vi "Example_Main.vi"() -> ()   [LabVIEW 2018, in "HttpExamples.lvlib"]
doc: "<b> </b> <b> </b>\nHttpClient_NET\nJustin Young - Viviota\nCopyright (c) 2021\nLicense: BSD"
uses:
  HttpExamples.lvlib
  Types/method_enum.ctl
  Types/ContentType.ctl
  <vilib>/Utility/sysdir.llb/System Directory Type.ctl
  HttpDownloadTask/HttpDownloadTask.lvclass/HttpDownloadTask.ctl
  HttpDownloadTask/Accessors/Read HttpResponseMessage.vi
  HttpContent_string/HttpContent_String.lvclass
  C:/Viviota/Projects/R&D/__OpenSource/VIV_HTTP_REST_NET/HttpContent/HttpContent.lvclass
  HttpHeaders_content/HttpHeaders_Content.lvclass
  C:/Viviota/Projects/R&D/__OpenSource/VIV_HTTP_REST_NET/HTTPHeaders_NET/HttpHeaders_NET.lvclass
  HttpHeaders_Request/HttpHeaders_Request.lvclass
  HttpHeaders_response/HttpHeaders_Response.lvclass
  <vilib>/httpClient/Base64Encode.vi
  HttpResponseMessage/HttpResponseMessage.lvclass
  HTTPHeaders_NET/HttpHeaders_NET.lvclass
  LabVIEWHTTPClient_NET/HttpClient_NET.lvclass
  WebProxy_NET/WebProxy_NET.lvclass
  HttpClient_NET.lvlib
  HttpRequestMessage/HttpRequestMessage.lvclass
  HttpContent_ByteArray/HttpContent_ByteArray.lvclass
  HttpContent_Stream/HttpContent_Stream.lvclass
  HttpContent_Multipart/HttpContent_Multipart.lvclass
  HttpContent/HttpContent.lvclass
  HttpDownloadTask/HttpDownloadTask.lvclass
panel:
  out "Error Out":errorcluster
  out "Status":u32
  in  "ExecutionExample":T1(ring)
  out "Header Values":string[](array[string])
  out "Header Names":string[](array[string])
  out "Response":string
  out "StatusCode":i32(ring)=100 items=["Continue"=100, "SwitchingProtocols"=101, "OK"=200, "Created"=201, "Accepted"=202, "NonAuthoritativeInformation"=203, "NoContent"=204, "ResetContent"=205, "PartialContent"=206, "MultipleChoices, Ambiguous"=300, "MovedPermanently, Moved"=301, "Found, Redirect"=302, "SeeOther, RedirectMethod"=303, "NotModified"=304, "UseProxy"=305, "Unused"=306, "TemporaryRedirect, RedirectKeepVerb"=307, "BadRequest"=400, "Unauthorized"=401, "PaymentRequired"=402, "Forbidden"=403, "NotFound"=404, "MethodNotAllowed"=405, "NotAcceptable"=406, "ProxyAuthenticationRequired"=407, "RequestTimeout"=408, "Conflict"=409, "Gone"=410, "LengthRequired"=411, "PreconditionFailed"=412, "RequestEntityTooLarge"=413, "RequestUriTooLong"=414, "UnsupportedMediaType"=415, "RequestedRangeNotSatisfiable"=416, "ExpectationFailed"=417, "UpgradeRequired"=426, "InternalServerError"=500, "NotImplemented"=501, "BadGateway"=502, "ServiceUnavailable"=503, "GatewayTimeout"=504, "HttpVersionNotSupported"=505]
  out "ReasonPhrase":string
  out "Timeout":bool
  in  "URL":string="https://reqres.in/api/users?page=2"
  in  "ProxyPort":i32=443
  in  "ProxyHost":string
  in  "UseProxy":bool
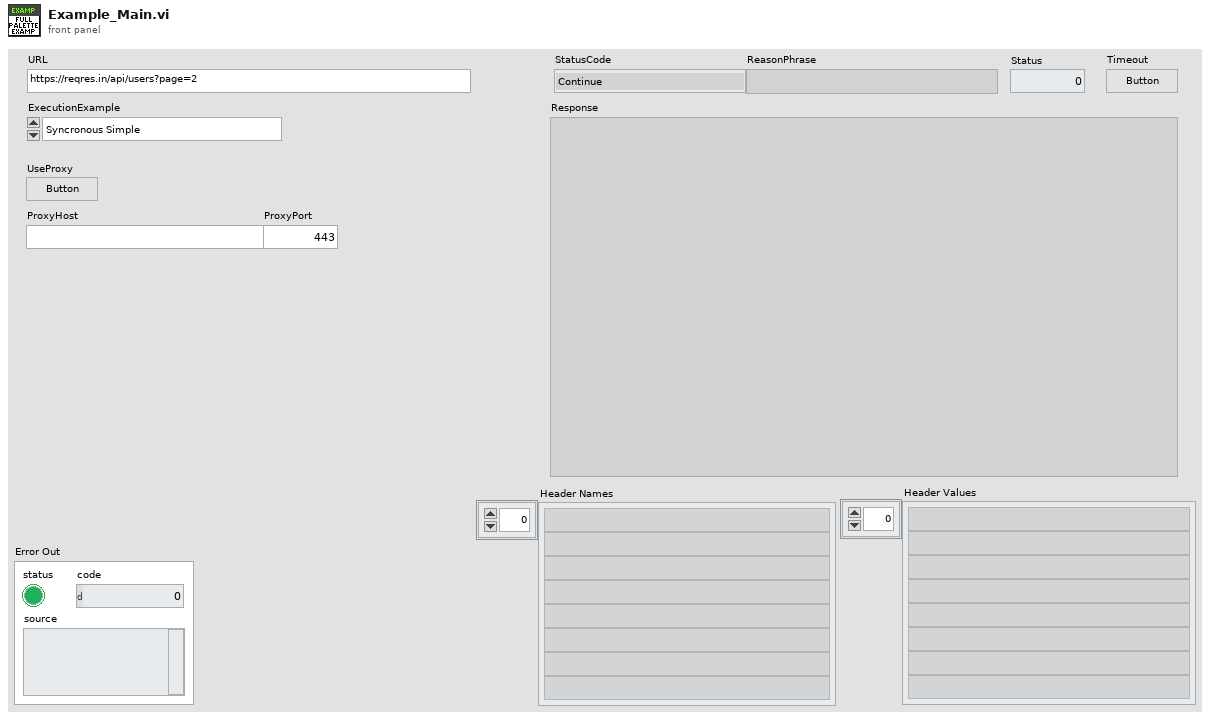
[diagram p1: front panel]
types:
  T1 = enum16{"Syncronous Simple", "Syncronous Advanced", "Asyncronous", "Asyncronous Queue", "Asyncronous File Download"}
  T2 = typedef "HttpClient_NET.lvlib/ContentType.ctl" = string
  T3 = enum16{"String", "ByteArray", "File", "MultiPart"}
  T4 = typedef "HttpClient_NET.lvlib/method_enum.ctl" = enum16{"GET", "PUT", "POST", "DELETE", "HEAD", "TRACE", "SEND"}
  T5 = typedef "HttpClient_NET.lvlib/ResponseHeaders_Cluster.ctl" = cluster{"ResponseHeader":refnum<class "HttpHeaders_Response.lvclass">, "ContentHeaders":refnum<class "HttpHeaders_Content.lvclass">}
  T6 = cluster{"HTTPHeaders_NET out":refnum<class "HttpHeaders_Response.lvclass">, "HTTPHeaders":refnum<class "HttpHeaders_Content.lvclass">}
  T7 = typedef "System Directory Type.ctl" = i32
  T8 = typedef "HttpClient_NET.lvlib/HttpDownloadTask.lvclass/DownloadTask_ref.ctl" = refnum<data-value>
  T9 = typedef "HttpClient_NET.lvlib/DownloadStats_Cluster.ctl" = cluster{"PositionCurrent":dbl, "PositionPrev":dbl, "TimeCurrent":timestamp, "TimePrev":timestamp, "TimeTotal":dbl, "PositionTotal":dbl, "TimeArray":dbl[], "PositionDifArray":dbl[], "CurrentRate":dbl, "RunningRate_10":dbl, "RunningRate":dbl, "Length":dbl}
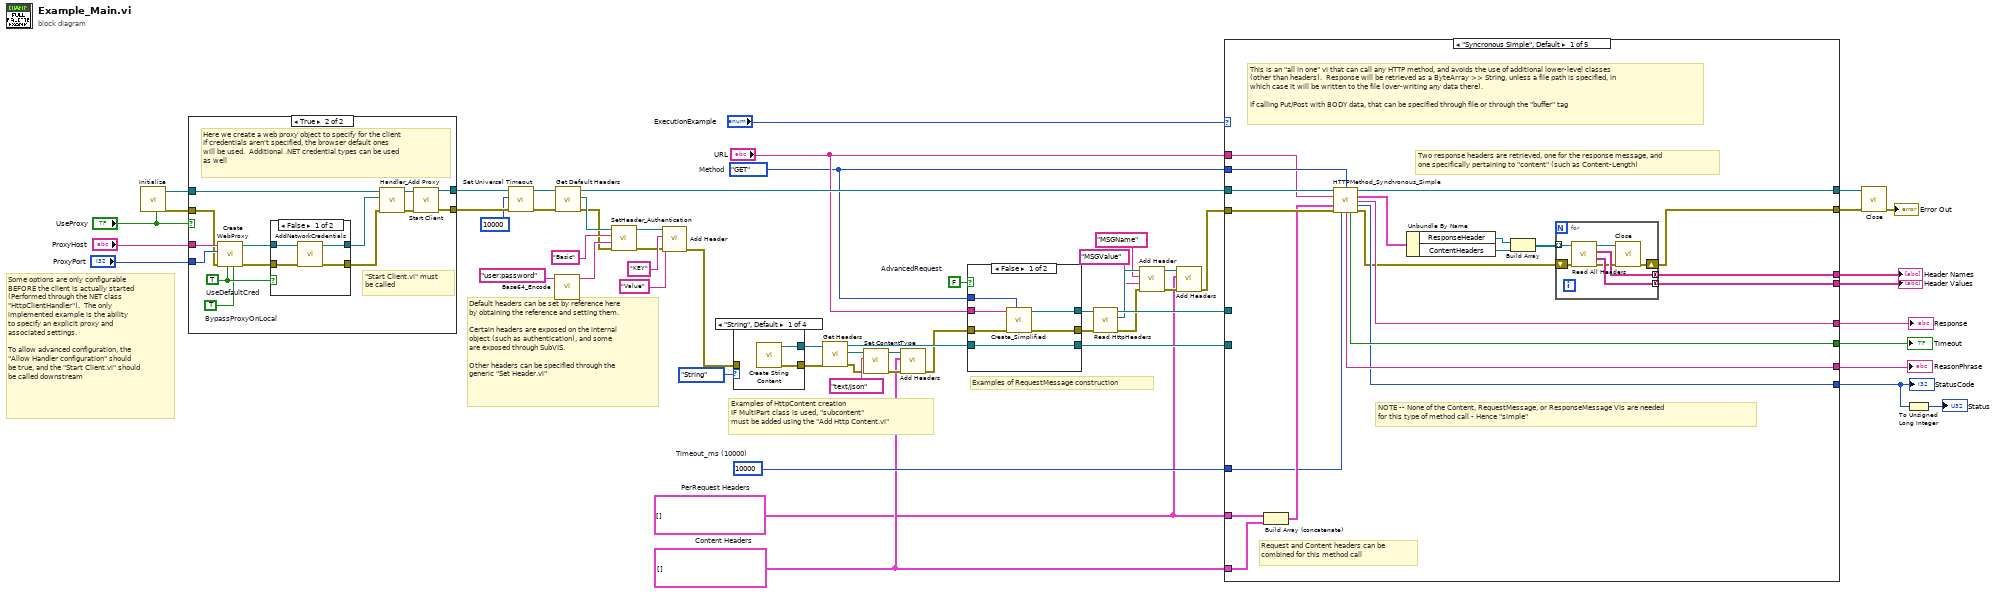
[diagram p0: block diagram]
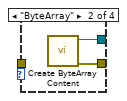
[diagram p4: hidden frame]
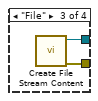
[diagram p5: hidden frame]
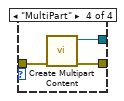
[diagram p6: hidden frame]
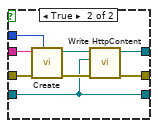
[diagram p7: hidden frame]
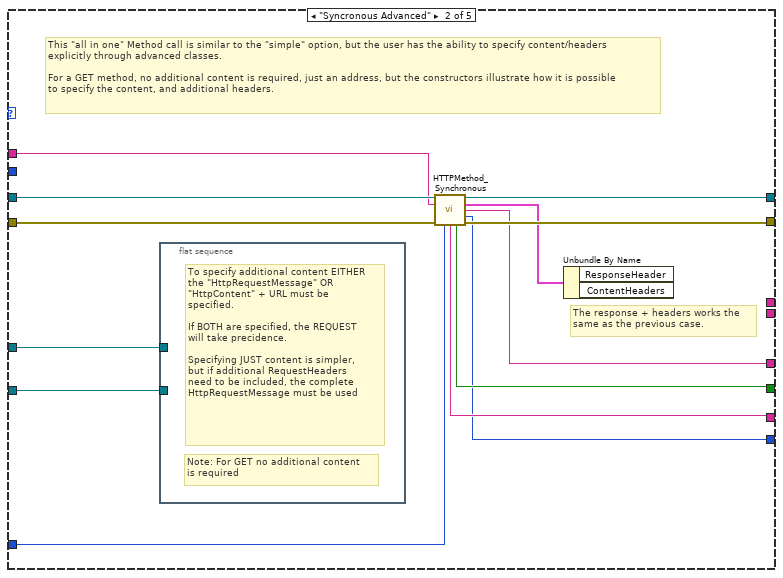
[diagram p8: hidden frame]
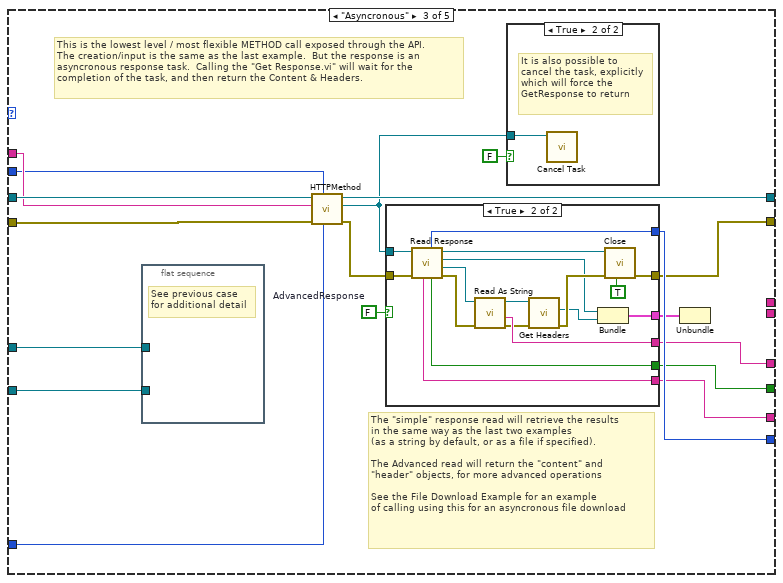
[diagram p9: hidden frame]
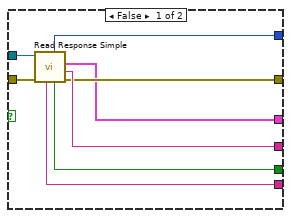
[diagram p11: hidden frame]
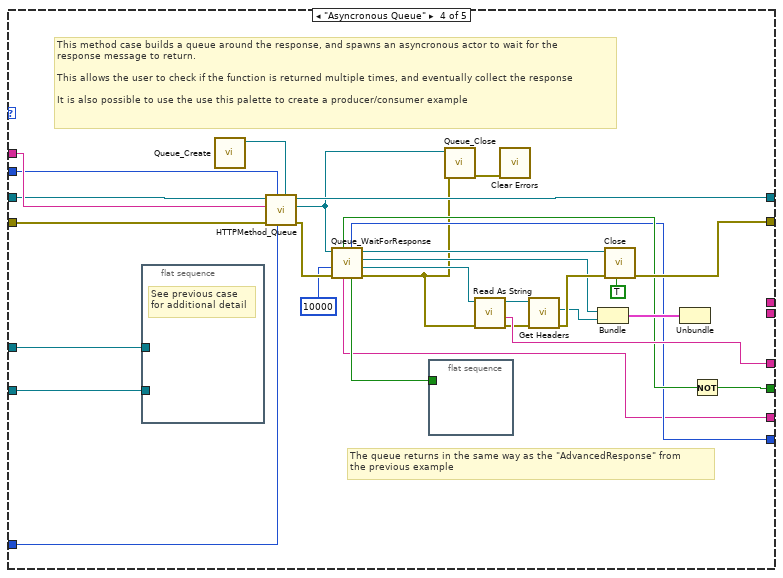
[diagram p12: hidden frame]
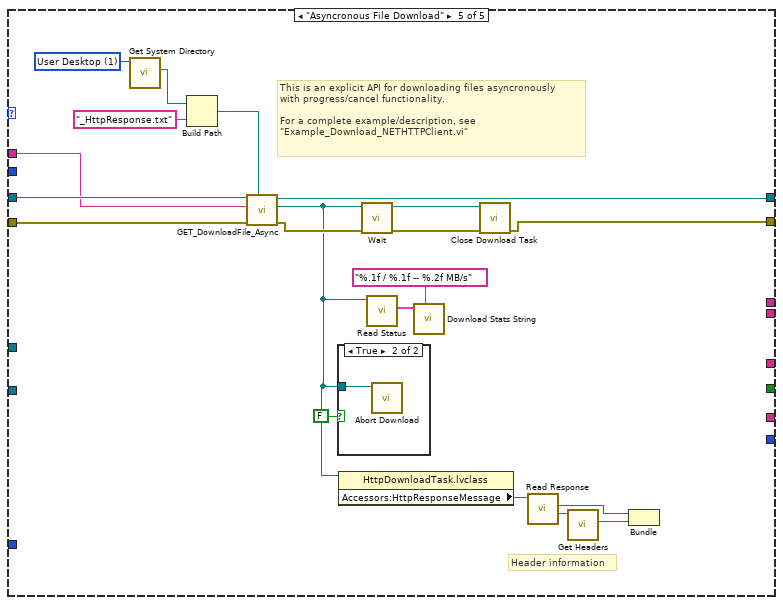
[diagram p13: hidden frame]
diagram:
  w12 = FALSE  # AdvancedRequest
  w38 = 10000  # Timeout_ms (10000)
  w5 = cluster{"header":string, "value":string}[] []  # Content Headers
  w4 = cluster{"header":string, "value":string}[] []  # PerRequest Headers
  w29 = method_enum."GET"  # Method
  # "Examples of HttpContent creation\nIF MultiPart class is used, \"subcontent\"\nmust be added using the \"Add Http Content.vi\""
  # "Examples of RequestMessage construction"
  # "Default headers can be set by reference here\nby obtaining the reference and setting them.\n\nCertain headers are exposed on the internal\nobject (such as authentication), and some\nare exposed through SubVIS.\n\nOther headers can be specified through the \ngeneric \"Set Header.vi\""
  # "Some options are only configurable\nBEFORE the client is actually started\n(Performed through the NET class\n\"HttpClientHandler\").  The only\nimplemented example is the ability\nto specify an explicit proxy and\nassociated settings.\n\nTo allow advanced configuration, the\n\"Allow Handler configuration\" should\nbe true, and the \"Start Client.vi\" should\nbe called downstream"
  n1 = call "Initialize.vi"("Allow Handler Configuration [F]"="UseProxy") -> ("error out"=w51:errorcluster, "HTTP Client Out"=w52:refnum<class "HttpClient_NET.lvclass">)  [unwired: 9 in]
  n2 = case shown="True" "UseProxy" {
    tunnel: w52 -> [w60 w75]
    tunnel: w51 -> [w61 w64]
    tunnel: [w60 w72] -> w50
    tunnel: [w61 w71] -> w49
    tunnel: "ProxyHost" -> [_ w70]
    tunnel: "ProxyPort" -> [_ w69]
    frame False {
      # "If the \"Allow Handler configuration\" is FALSE, then \nthe start client.vi does not need to be called explicitly"
    }
    frame True {
      w62 = TRUE  # BypassProxyOnLocal
      w63 = TRUE  # UseDefaultCred
      # "\"Start Client.vi\" must\nbe called"
      # "Here we create a web proxy object to specify for the client\nIf credentials aren't specified, the browser default ones\nwill be used.  Additional .NET credential types can be used\nas well"
      n3 = call "Create WebProxy.vi"("BypassProxyOnLocal"=w62, "UseDefaultCredentials [T]"=w63, "Error In"=w64, "Port (443)"=w69, "Host"=w70) -> ("Error Out"=w66:errorcluster, "WebProxy Out"=w68:refnum<class "WebProxy_NET.lvclass">)  [unwired: 5 in]
      n4 = case shown="False" w63 {
        tunnel: w68 -> [w79 w81]
        tunnel: [w78 w81] -> w67
        tunnel: w66 -> [w77 w80]
        tunnel: [w76 w80] -> w65
        frame False {
          n5 = call "AddNetworkCredentials.vi"("error in (no error)"=w77, "WebProxy_NET in"=w79) -> ("error out"=w76:errorcluster, "WebProxy_NET out"=w78:refnum<class "WebProxy_NET.lvclass">)  [unwired: 8 in]
        }
        frame True {
        }
      }
      n6 = call "Handler_Add Proxy.vi"("error in (no error)"=w65, "WebProxy"=w67, "LabVIEWHTTPClient_NET in"=w75) -> ("error out"=w73:errorcluster, "LabVIEWHTTPClient_NET out"=w74:refnum<class "HttpClient_NET.lvclass">)  [unwired: 7 in]
      n7 = call "Start Client.vi"("error in (no error)"=w73, "LabVIEWHTTPClient_NET in"=w74) -> ("error out"=w71:errorcluster, "LabVIEWHTTPClient_NET out"=w72:refnum<class "HttpClient_NET.lvclass">)  [unwired: 8 in]
    }
  }
  n8 = call "Set Universal Timeout.vi"("error in (no error)"=w49, "timeout_ms (10000)"=10000, "LabVIEWHTTPClient_NET in"=w50) -> ("error out"=w59:errorcluster, "LabVIEWHTTPClient_NET out"=w58:refnum<class "HttpClient_NET.lvclass">)  [unwired: 7 in]
  n9 = call "Base64_Encode.vi"("buffer in"="user:password" ("scheme")) -> ("encoded string"=w54:string)  [unwired: 5 in, 1 out]
  n10 = call "Get Default Headers.vi"("error in (no error)"=w59, "LabVIEWHTTPClient_NET in"=w58) -> ("error out"=w53:errorcluster, "DefaultRequest Headers"=w57:refnum<class "HttpHeaders_Request.lvclass">, "LabVIEWHTTPClient_NET out"=w39:refnum<class "HttpClient_NET.lvclass">)  [unwired: 7 in]
  n11 = call "SetHeader_Authentication.vi"("error in (no error)"=w53, "parameter"=w54, "scheme"="Basic", "HttpHeaders_Request in"=w57) -> ("error out"=w41:errorcluster, "HttpHeaders_Request out"=w42:refnum<class "HttpHeaders_Request.lvclass">)  [unwired: 6 in]
  n12 = call-dynamic "Add Header.vi"("error in (no error)"=w41, "Value"="Value", "Name"="KEY", "HTTPHeaders_NET in"=w42) -> ("error out"=w27:errorcluster)  [unwired: 6 in, 1 out]
  n13 = case shown="\"String\", Default" T3."String" {
    tunnel: [w83 w85 w86 w89] -> w25
    tunnel: [w82 w84 w87 w90] -> w26
    tunnel: w27 -> [_ _ _ w88]
    frame "String", Default {
      n14 = call "Create String Content.vi"() -> ("error out"=w82:errorcluster, "HttpContent_String out"=w83:refnum<class "HttpContent_String.lvclass">)  [unwired: 10 in]
    }
    frame "ByteArray" {
      n15 = call "Create ByteArray Content.vi"() -> ("error out"=w84:errorcluster, "HttpContent_String out"=w85:refnum<class "HttpContent_ByteArray.lvclass">)  [unwired: 10 in]
    }
    frame "File" {
      n16 = call "Create File Stream Content.vi"() -> ("error out"=w87:errorcluster, "HttpContent_Stream out"=w86:refnum<class "HttpContent_Stream.lvclass">)  [unwired: 10 in]
    }
    frame "MultiPart" {
      n17 = call "Create Multipart Content.vi"("error in (no error)"=w88) -> ("error out"=w90:errorcluster, "HttpContent_Multipart out"=w89:refnum<class "HttpContent_Multipart.lvclass">)  [unwired: 9 in]
    }
  }
  n18 = call "Get Headers.vi"("error in (no error)"=w26, "HttpContent in"=w25) -> ("error out"=w22:errorcluster, "HTTPHeaders"=w24:refnum<class "HttpHeaders_Content.lvclass">, "HttpContent out"=w21:refnum<class "HttpContent.lvclass">)  [unwired: 7 in]
  n19 = call "Set ContentType.vi"("error in (no error)"=w22, "ContentType"=T2 "text/json", "HttpHeaders_Content in"=w24) -> ("error out"=w7:errorcluster, "HttpHeaders_Content out"=w8:refnum<class "HttpHeaders_Content.lvclass">)  [unwired: 7 in]
  n20 = call "Add Headers.vi"("error in (no error)"=w7, "headers"=w5, "HttpHeaders_NET in"=w8) -> ("error out"=w6:errorcluster)  [unwired: 7 in, 1 out]
  n21 = case shown="False" w12 {
    tunnel: [w93 w103] -> w19
    tunnel: [w92 w102] -> w18
    tunnel: "URL" -> [w95 w100]
    tunnel: w29 -> [w94 w99]
    tunnel: w6 -> [w96 w98]
    tunnel: w21 -> [w91 w97]
    tunnel: [w91 w97] -> w20
    frame False {
      n22 = call "Create_Simplified.vi"("Method [GET]"=w94, "error in (no error)"=w96, "Address"=w95) -> ("error out"=w92:errorcluster, "HttpRequestMessage out"=w93:refnum<class "HttpRequestMessage.lvclass">)  [unwired: 6 in, 1 out]
    }
    frame True {
      n23 = call "Create.vi"("Method [GET]"=w99, "error in (no error)"=w98, "Address"=w100) -> ("error out"=w101:errorcluster, "HttpRequestMessage out"=w104:refnum<class "HttpRequestMessage.lvclass">)  [unwired: 7 in]
      n24 = call "Write HttpContent.vi"("error in (no error)"=w101, "HttpContent"=w97, "HttpRequestMessage in"=w104) -> ("error out"=w102:errorcluster, "HttpRequestMessage out"=w103:refnum<class "HttpRequestMessage.lvclass">)  [unwired: 7 in]
    }
  }
  n25 = call "Read HttpHeaders.vi"("error in (no error)"=w18, "HttpRequestMessage in"=w19) -> ("error out"=w13:errorcluster, "HttpHeaders"=w16:refnum<class "HttpHeaders_Request.lvclass">, "HttpRequestMessage out"=w17:refnum<class "HttpRequestMessage.lvclass">)  [unwired: 7 in]
  n26 = call-dynamic "Add Header.vi"("error in (no error)"=w13, "Value"="MSGValue", "Name"="MSGName", "HTTPHeaders_NET in"=w16) -> ("error out"=w10:errorcluster, "HTTPHeaders_NET out"=w11:refnum<class "HttpHeaders_Request.lvclass">)  [unwired: 6 in]
  n27 = call "Add Headers.vi"("error in (no error)"=w10, "headers"=w4, "HttpHeaders_NET in"=w11) -> ("error out"=w9:errorcluster)  [unwired: 7 in, 1 out]
  n28 = case shown="\"Syncronous Simple\", Default" "ExecutionExample" {
    tunnel: w9 -> [w125 w144 w161 w214 w239]
    tunnel: w39 -> [w124 w145 w160 w212 w238]
    tunnel: "URL" -> [w122 w142 w159 w213 w237]
    tunnel: w29 -> [w123 _ w157 w209 _]
    tunnel: w4 -> [w121 _ _ _ _]
    tunnel: w5 -> [w120 _ _ _ _]
    tunnel: w38 -> [w118 w139 w158 w210 _]
    tunnel: [w117 w137 w152 w198 _] -> w37
    tunnel: [w116 w138 w153 w194 _] -> w36
    tunnel: [w115 w134 w154 w197 _] -> w3
    tunnel: [w114 w135 w151 w217 _] -> w35
    tunnel: [w108 _ _ _ _] -> w34
    tunnel: [w107 _ _ _ _] -> w33
    tunnel: [w106 w143 w155 w211 w225] -> w32
    tunnel: [w105 w136 w150 w216 w226] -> w31
    tunnel: w20 -> [_ w141 w163 w219 _]
    tunnel: w17 -> [_ w140 w162 w218 _]
    frame "Syncronous Simple", Default {
      # "NOTE -- None of the Content, RequestMessage, or ResponseMessage VIs are needed\nfor this type of method call - Hence \"simple\""
      # "Request and Content headers can be\ncombined for this method call"
      # "Two response headers are retrieved, one for the response message, and\none specifically pertaining to \"content\" (such as Content-Length)"
      # "This is an \"all in one\" vi that can call any HTTP method, and avoids the use of additional lower-level classes\n(other than headers).  Response will be retrieved as a ByteArray >> String, unless a file path is specified, in\nwhich case it will be written to the file (over-writing any data there).\n\nIf calling Put/Post with BODY data, that can be specified through file or through the \"buffer\" tag"
      n29 = Build Array (concatenate)(w121, w120) -> (w119:cluster{"header":string, "value":string}[])
      n30 = call "HTTPMethod_Synchronous_Simple.vi"("LabVIEWHTTPClient_NET in"=w124, "Method"=w123, "URL"=w122, "request headers"=w119, "error in (no error)"=w125, "Timeout_ms (10000)"=w118) -> ("LabVIEWHTTPClient_NET out"=w106:refnum<class "HttpClient_NET.lvclass">, "Headers"=w113:T5, "Response"=w114:string, "StatusCode"=w115:i32, "ReasonPhrase"=w116:string, "Timeout"=w117:bool, "error out"=w109:errorcluster)  [unwired: 3 in]
      n31 = Unbundle By Name(w113) -> ("ResponseHeader"=w112:refnum<class "HttpHeaders_Response.lvclass">, "ContentHeaders"=w111:refnum<class "HttpHeaders_Content.lvclass">)
      n32 = Build Array(w112, w111) -> (w110:refnum<class "HttpHeaders_NET.lvclass">[])
      n33 = for {
        tunnel: w110 -> [w132] mode=indexing
        tunnel: [w131] -> w108 mode=concatenating
        tunnel: [w130] -> w107 mode=concatenating
        shift-right: [w127] -> w105
        shift-left: w109 -> [w129]
        n34 = call-dynamic "Read All Headers.vi"("error in (no error)"=w129, "HTTPHeaders_NET in"=w132) -> ("error out"=w128:errorcluster, "Header Values"=w130:string[], "Header Names"=w131:string[], "HTTPHeaders_NET out"=w126:refnum<class "HttpHeaders_NET.lvclass">)  [unwired: 6 in]
        n35 = call "Close.vi"("error in (no error)"=w128, "HTTPHeaders_NET in"=w126) -> ("error out"=w127:errorcluster)  [unwired: 9 in]
      }
    }
    frame "Syncronous Advanced" {
      # "The response + headers works the \nsame as the previous case."
      # "This \"all in one\" Method call is similar to the \"simple\" option, but the user has the ability to specify content/headers\nexplicitly through advanced classes.\n\nFor a GET method, no additional content is required, just an address, but the constructors illustrate how it is possible\nto specify the content, and additional headers."
      n36 = flat-sequence {
        tunnel: w141 -> [_]
        tunnel: w140 -> [_]
        frame #0 {
          # "Note: For GET no additional content\nis required"
          # "To specify additional content EITHER\nthe \"HttpRequestMessage\" OR\n\"HttpContent\" + URL must be\nspecified.\n\nIf BOTH are specified, the REQUEST \nwill take precidence.\n\nSpecifying JUST content is simpler, \nbut if additional RequestHeaders\nneed to be included, the complete\nHttpRequestMessage must be used"
        }
      }
      n37 = call "HTTPMethod_Synchronous.vi"("LabVIEWHTTPClient_NET in"=w145, "URL"=w142, "error in (no error)"=w144, "Timeout_ms (10000)"=w139) -> ("LabVIEWHTTPClient_NET out"=w143:refnum<class "HttpClient_NET.lvclass">, "Headers"=w133:T5, "Response"=w135:string, "StatusCode"=w134:i32, "ReasonPhrase"=w138:string, "Timeout"=w137:bool, "error out"=w136:errorcluster)  [unwired: 5 in]
      n38 = Unbundle By Name(w133) -> ()  [unwired: 2 out]
    }
    frame "Asyncronous" {
      w148 = FALSE  # AdvancedResponse
      # "The \"simple\" response read will retrieve the results\nin the same way as the last two examples \n(as a string by default, or as a file if specified).\n\nThe Advanced read will return the \"content\" and\n\"header\" objects, for more advanced operations \n\nSee the File Download Example for an example\nof calling using this for an asyncronous file download"
      # "This is the lowest level / most flexible METHOD call exposed through the API.\nThe creation/input is the same as the last example.  But the response is an \nasyncronous response task.  Calling the \"Get Response.vi\" will wait for the\ncompletion of the task, and then return the Content & Headers."
      n39 = flat-sequence {
        tunnel: w162 -> [_]
        tunnel: w163 -> [_]
        frame #0 {
          # "See previous case\nfor additional detail"
        }
      }
      n40 = call "HTTPMethod.vi"("Timeout_ms (10000)"=w158, "Method"=w157, "error in (no error)"=w161, "URL"=w159, "LabVIEWHTTPClient_NET in"=w160) -> ("error out"=w156:errorcluster, "HttpResponseMessage out"=w147:refnum<class "HttpResponseMessage.lvclass">, "LabVIEWHTTPClient_NET out"=w155:refnum<class "HttpClient_NET.lvclass">)  [unwired: 4 in]
      n41 = case shown="True" w148 {
        tunnel: w156 -> [w172 w189]
        tunnel: w147 -> [w171 w188]
        tunnel: [w168 w187] -> w154
        tunnel: [w170 w186] -> w153
        tunnel: [w169 w185] -> w152
        tunnel: [w167 w182] -> w151
        tunnel: [w166 w184] -> w150
        tunnel: [w165 w174] -> w149
        frame False {
          n42 = call "Read Response Simple.vi"("error in (no error)"=w172, "HttpResponseMessage in"=w171) -> ("error out"=w166:errorcluster, "Response"=w167:string, "Headers"=w165:T5, "Timeout"=w169:bool, "StatusCode"=w168:i32, "ReasonPhrase"=w170:string)  [unwired: 4 in]
        }
        frame True {
          n43 = call "Read Response.vi"("error in (no error)"=w189, "HttpResponseMessage in"=w188) -> ("error out"=w179:errorcluster, "HttpContent out"=w183:refnum<class "HttpContent.lvclass">, "HTTPHeaders_NET out"=w175:refnum<class "HttpHeaders_Response.lvclass">, "HttpResponseMessage out"=w173:refnum<class "HttpResponseMessage.lvclass">, "Timeout"=w185:bool, "StatusCode"=w187:i32, "ReasonPhrase"=w186:string)  [unwired: 3 in]
          n44 = call "Read As String.vi"("error in (no error)"=w179, "HttpContent in"=w183) -> ("error out"=w181:errorcluster, "Content"=w182:string, "HttpContent out"=w178:refnum<class "HttpContent.lvclass">)  [unwired: 7 in]
          n45 = call "Get Headers.vi"("error in (no error)"=w181, "HttpContent in"=w178) -> ("error out"=w177:errorcluster, "HTTPHeaders"=w176:refnum<class "HttpHeaders_Content.lvclass">)  [unwired: 7 in, 1 out]
          n46 = Bundle("HTTPHeaders_NET out"=w175, "HTTPHeaders"=w176) -> (w174:T6)  [unwired: 1 in]
          n47 = call "Close.vi"("CloseHeaders"=TRUE, "error in (no error)"=w177, "HttpResponseMessage in"=w173) -> ("error out"=w184:errorcluster)  [unwired: 8 in]
        }
      }
      n48 = case shown="True" FALSE {
        tunnel: w147 -> [_ w164]
        frame False {
        }
        frame True {
          # "It is also possible to \ncancel the task, explicitly\nwhich will force the\nGetResponse to return"
          n49 = call "Cancel Task.vi"("HttpResponseMessage in"=w164) -> ()  [unwired: 9 in, 2 out]
        }
      }
      n50 = Unbundle(w149) -> ()  [unwired: 2 out]
    }
    frame "Asyncronous Queue" {
      # "The queue returns in the same way as the \"AdvancedResponse\" from\nthe previous example"
      # "This method case builds a queue around the response, and spawns an asyncronous actor to wait for the\nresponse message to return.\n\nThis allows the user to check if the function is returned multiple times, and eventually collect the response\n\nIt is also possible to use the use this palette to create a producer/consumer example"
      n51 = flat-sequence {
        tunnel: w218 -> [_]
        tunnel: w219 -> [_]
        frame #0 {
          # "See previous case\nfor additional detail"
        }
      }
      n52 = call "Queue_Create.vi"() -> ("Queue out"=w193:refnum<queue>)  [unwired: 10 in, 1 out]
      n53 = call "HTTPMethod_Queue.vi"("Queue In [create if empty]"=w193, "Timeout_ms (10000)"=w210, "Method"=w209, "error in (no error)"=w214, "URL"=w213, "LabVIEWHTTPClient_NET in"=w212) -> ("error out"=w208:errorcluster, "Queue Out"=w191:refnum<queue>, "LabVIEWHTTPClient_NET out"=w211:refnum<class "HttpClient_NET.lvclass">)  [unwired: 3 in]
      n54 = call "Queue_WaitForResponse.vi"("error in (no error)"=w208, "QueueTimeout_ms (10000)"=10000, "Response Queue"=w191) -> ("error out"=w192:errorcluster, "HttpContent out"=w202:refnum<class "HttpContent.lvclass">, "HTTPHeaders_NET out"=w201:refnum<class "HttpHeaders_Response.lvclass">, "HttpResponseMessage out"=w200:refnum<class "HttpResponseMessage.lvclass">, "Queue timed out?"=w196:bool, "StatusCode"=w197:i32, "ReasonPhrase"=w194:string, "TaskSuccess"=w199:bool)  [unwired: 1 in]
      n55 = flat-sequence {
        tunnel: w196 -> [_]
        frame #0 {
        }
      }
      n56 = call "Queue_Close.vi"("Error In"=w192, "Response Queue"=w191) -> ("Error Out"=w190:errorcluster)  [unwired: 9 in]
      n57 = call "Read As String.vi"("error in (no error)"=w192, "HttpContent in"=w202) -> ("error out"=w207:errorcluster, "Content"=w217:string, "HttpContent out"=w205:refnum<class "HttpContent.lvclass">)  [unwired: 7 in]
      n58 = call <vilib>:"Clear Errors.vi"("error in (no error)"=w190) -> ()  [unwired: 5 in, 2 out]
      n59 = call "Get Headers.vi"("error in (no error)"=w207, "HttpContent in"=w205) -> ("error out"=w204:errorcluster, "HTTPHeaders"=w203:refnum<class "HttpHeaders_Content.lvclass">)  [unwired: 7 in, 1 out]
      n60 = Bundle("HTTPHeaders_NET out"=w201, "HTTPHeaders"=w203) -> (w215:T6)  [unwired: 1 in]
      n61 = call "Close.vi"("CloseHeaders"=TRUE, "error in (no error)"=w204, "HttpResponseMessage in"=w200) -> ("error out"=w216:errorcluster)  [unwired: 8 in]
      n62 = Unbundle(w215) -> ()  [unwired: 2 out]
      n63 = Not(x=w199) -> (.not. x?=w198:bool)
    }
    frame "Asyncronous File Download" {
      w236 = T7 1 items=["User Home"=0, "User Desktop"=1, "User Documents"=2, "User Application Data"=3, "User Preferences"=4, "User Temporary"=5, "Public Documents"=6, "Public Application Data"=7, "Public Preferences"=8, "Public Cache"=13, "System Core Libraries"=9, "System Installed Libraries"=10, "Application Files"=11, "Boot Volume Root"=12] ("system directory type")
      # "Header information"
      # "This is an explicit API for downloading files asyncronously\nwith progress/cancel functionality.\n\nFor a complete example/description, see \n\"Example_Download_NETHTTPClient.vi\""
      n64 = call <vilib>:"Get System Directory.vi"("system directory type"=w236) -> ("system directory"=w235:path)  [unwired: 10 in]
      n65 = Build Path(base path=w235, name or relative path="_HttpResponse.txt") -> (appended path=w233:path)
      n66 = call "GET_DownloadFile_Async.vi"("TargetFilePath"=w233, "error in (no error)"=w239, "URL"=w237, "LabVIEWHTTPClient_NET in"=w238) -> ("error out"=w228:errorcluster, "DownloadTask Ref"=w224:T8, "LabVIEWHTTPClient_NET out"=w225:refnum<class "HttpClient_NET.lvclass">)  [unwired: 5 in]
      n67 = case shown="True" FALSE {
        tunnel: w224 -> [_ w240]
        frame False {
        }
        frame True {
          n68 = call "Abort Download.vi"("HttpDownloadTask in"=w240) -> ()  [unwired: 9 in, 2 out]
        }
      }
      n69 = property class="HttpDownloadTask.lvclass"(reference=w224) -> ("Accessors:HttpResponseMessage"=w222:refnum<class "HttpResponseMessage.lvclass">)  [unwired: 1 in, 2 out]
      n70 = call "Wait.vi"("error in (no error)"=w228, "HttpDownloadTask in"=w224) -> ("error out"=w227:errorcluster, "HttpDownloadTask out"=w232:T8)  [unwired: 6 in, 2 out]
      n71 = call "Read Status.vi"("HttpDownloadTask in"=w224) -> ("RunningStats"=w230:T9)  [unwired: 6 in, 4 out]
      n72 = call "Download Stats String.vi"("Format String (3 floats)"="%.1f / %.1f -- %.2f MB/s" ("format string"), "Status Cluster"=w230) -> ()  [unwired: 8 in, 2 out]
      n73 = call "Close Download Task.vi"("error in (no error)"=w227, "HttpDownloadTask in"=w232) -> ("error out"=w226:errorcluster)  [unwired: 9 in]
      n74 = call "Read Response.vi"("HttpResponseMessage in"=w222) -> ("HttpContent out"=w220:refnum<class "HttpContent.lvclass">, "HTTPHeaders_NET out"=w221:refnum<class "HttpHeaders_Response.lvclass">)  [unwired: 4 in, 5 out]
      n75 = call "Get Headers.vi"("HttpContent in"=w220) -> ("HTTPHeaders"=w223:refnum<class "HttpHeaders_Content.lvclass">)  [unwired: 8 in, 2 out]
      n76 = Bundle("HTTPHeaders_NET out"=w221, "HTTPHeaders"=w223) -> ()  [unwired: 1 in, 1 out]
    }
  }
  "Timeout" <- w37
  "ReasonPhrase" <- w36
  "StatusCode" <- w3
  "Response" <- w35
  "Header Names" <- w34
  "Header Values" <- w33
  n77 = call "Close.vi"("Error In"=w31, "LabVIEWHTTPClient_NET in"=w32) -> ("Error Out"=→"Error Out":errorcluster)  [unwired: 9 in]
  n78 = To Unsigned Long Integer(number=w3) -> (unsigned 32bit integer=→"Status":u32)
